vi "HumanGlobal.vi"() -> ()   [LabVIEW 2023]
uses:
  HumanDriveModeENUM.ctl
panel:
  out "Human_DriveFIeldOriented":bool
  out "Human_DriveMode":T1
  out "AutoSpeakerAngleEnabled":bool
  out "InsideWingX":bool
  out "InRange":bool
  out "OnTargetSpeaker":bool
  out "DesiredAngularSpeed (degree/s)":dbl
  out "DesiredAngleToSpeaker (degrees)":dbl
  out "DistanceToSpeaker (m)":dbl
  out "ReverseX":bool
  out "StateChangeX":bool
  out "DPadLeftZ":bool
  out "DPadRightZ":bool
  out "DPadDownZ":bool
  out "DPadUpZ":bool
  # "UNUSED"
  # "VISION TARGETTING"
  # "DRIVING MODES"
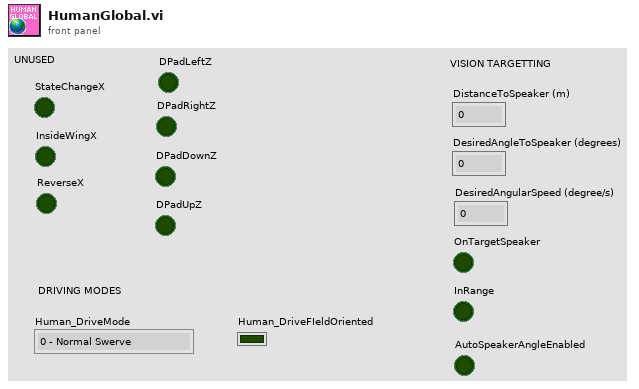
[diagram p1: front panel]
types:
  T1 = typedef "HumanDriveModeENUM.ctl" = enum16{"0 - Normal Swerve", "1 - Auto traj  - Left Speaker", "2 - Auto traj - Center Speaker", "3 - Auto traj - Speaker Right", "4 - Auto traj - Amp", "5 - Auto traj - Source", "6 - Auto traj -  Left Stage", "7 - Auto traj - Center Stage", "8 - Auto traj - Right Stage"}
diagram:
